vi "PathPlanner_Cmd_Follow_Internal_Replan_Sample.vi"(4 "PassthroughTime_SEC":dbl, 5 "Extra Time Sec":dbl, 6 "Reset In":bool, 7 "ReplanningConfig":T6={"enableInitialReplanning"=TRUE, "enableDynamicReplanning"=FALSE, "dynamicReplanningTotalErrorThreshold"=1.0, "dynamicReplanningErrorSpikeThreshold"=0.25}, 8 "Position Error M":dbl, 9 "Current Pose SI":T17 {"ROTATION"."SIN" format="%13.4f"; "ROTATION"."COS" format="%13.4f"; "ROTATION"."VALUE" format="%13.4f"; "TRANSLATION"."Y" format="%14.3f"; "TRANSLATION"."X" format="%14.3f"}, 10 "CurrentChassisSpeeds":T18 {"vOmega" format="%10.3f"; "vY" format="%10.3f"; "vX" format="%10.3f"}, 11 "RePlannedPath in":T11 {"AllPoints"."HolonomicRotation"."SIN" format="%13.4f"; "AllPoints"."HolonomicRotation"."COS" format="%13.4f"; "AllPoints"."HolonomicRotation"."VALUE" format="%13.4f"; "AllPoints"."Position"."Y" format="%14.3f"; "AllPoints"."Position"."X" format="%14.3f"; "GoalEndState"."Rotation"."SIN" format="%13.4f"; "GoalEndState"."Rotation"."COS" format="%13.4f"; "GoalEndState"."Rotation"."VALUE" format="%13.4f"; "RotationTargets"."target"."SIN" format="%13.4f"; "RotationTargets"."target"."COS" format="%13.4f"; "RotationTargets"."target"."VALUE" format="%13.4f"; "PreviewStartingRotation"."SIN" format="%13.4f"; "PreviewStartingRotation"."COS" format="%13.4f"; "PreviewStartingRotation"."VALUE" format="%13.4f"; "BezierPoints"."Y" format="%14.3f"; "BezierPoints"."X" format="%14.3f"}) -> (0 "Traj End Status":T5, 1 "Trajectory State":T7={"TimeSeconds"=0.0, "VelocityMPS"=0.0, "AccerationMpsSq"=0.0, "HeadingAngularVelRadPerSec"=0.0, "PositionMeters"={"X"=0.0, "Y"=0.0}, "Heading"={"VALUE"=0.0, "COS"=1.0, "SIN"=0.0}, "TargetHolonomicRotation"={"VALUE"=0.0, "COS"=1.0, "SIN"=0.0}, "CurvatureRadPerMeter"=0.0, "PathPlannerConstraints"={"MaxVelocityMps;"=0.0, "MaxAccelerationMpsSq;"=0.0, "MaxAngularVelRadPsEc;"=0.0, "MaxAngularAccRadPSecSq"=0.0, "Exists"=FALSE}, "DeltaPos"=0.0} {"TargetHolonomicRotation"."SIN" format="%13.4f"; "TargetHolonomicRotation"."COS" format="%13.4f"; "TargetHolonomicRotation"."VALUE" format="%13.4f"; "Heading"."SIN" format="%13.4f"; "Heading"."COS" format="%13.4f"; "Heading"."VALUE" format="%13.4f"; "PositionMeters"."Y" format="%14.3f"; "PositionMeters"."X" format="%14.3f"}, 2 "Reset Controller":bool, 3 "PathPlannerTrajectoryEvents":T1)   [LabVIEW 2019, in "PathPlanner24.lvlib"]
doc: "This is an internal function. It is not to be called by end users."
uses:
  PathPlanner24.lvlib
  <vilib>/Rock Robotics/WPI/ThirdParty/JAS_Junk/TrajLib/TypeDef/CHASSIS_SPEEDS.ctl
  TypeDef/PathPlannerPath.ctl
  <vilib>/Rock Robotics/WPI/ThirdParty/JAS_Junk/TrajLib/TypeDef/TRANSLATION2D.ctl
  <vilib>/Rock Robotics/WPI/ThirdParty/JAS_Junk/TrajLib/TypeDef/ROTATION2D.ctl
  TypeDef/PathPlannerRotationTarget.ctl
  TypeDef/PathPlannerConstraintsZone.ctl
  TypeDef/PathPlannerPathConstraints.ctl
  TypeDef/PathPlannerEventMarker.ctl
  TypeDef/PathPlannerCommandUtil.ctl
  ENum/PathPlanner_CommandUtilType_ENUM.ctl
  TypeDef/PathPlannerGoalEndState.ctl
  TypeDef/PathPlannerPathPoint.ctl
  <vilib>/Rock Robotics/WPI/ThirdParty/JAS_Junk/TrajLib/TypeDef/POSE2D.ctl
  TypeDef/PathPlannerTrajectoryState.ctl
  TypeDef/PathPlannerReplanningConfig.ctl
  <vilib>/Rock Robotics/WPI/ThirdParty/JAS_Junk/TrajLib/Rotation2d_GetDegrees.vi
  <vilib>/Rock Robotics/WPI/ThirdParty/JAS_Junk/TrajLib/MathUtil_InputModulus.vi
  <vilib>/Rock Robotics/WPI/ThirdParty/JAS_Junk/TrajLib/Rotation2d_CreateAngleDegrees.vi
  <vilib>/Rock Robotics/WPI/ThirdParty/JAS_Junk/TrajLib/Rotation2d_GetRadians.vi
  <vilib>/Rock Robotics/WPI/ThirdParty/JAS_Junk/TrajLib/Conv_Radians_Deg.vi
  <vilib>/Rock Robotics/WPI/ThirdParty/JAS_Junk/TrajLib/Conv_Deg_Radians.vi
  <vilib>/Rock Robotics/WPI/ThirdParty/JAS_Junk/TrajLib/Rotation2d_CreateAngle.vi
  <vilib>/Utility/semaphor.llb/Obtain Semaphore Reference.vi
  <vilib>/Rock Robotics/WPI/ThirdParty/JAS_Junk/TrajLib/Trajectory_Library.lvlib
  TypeDef/PathPlannerTrajectoryEvent.ctl
  TypeDef/PathPlannerTrajectoryEvents.ctl
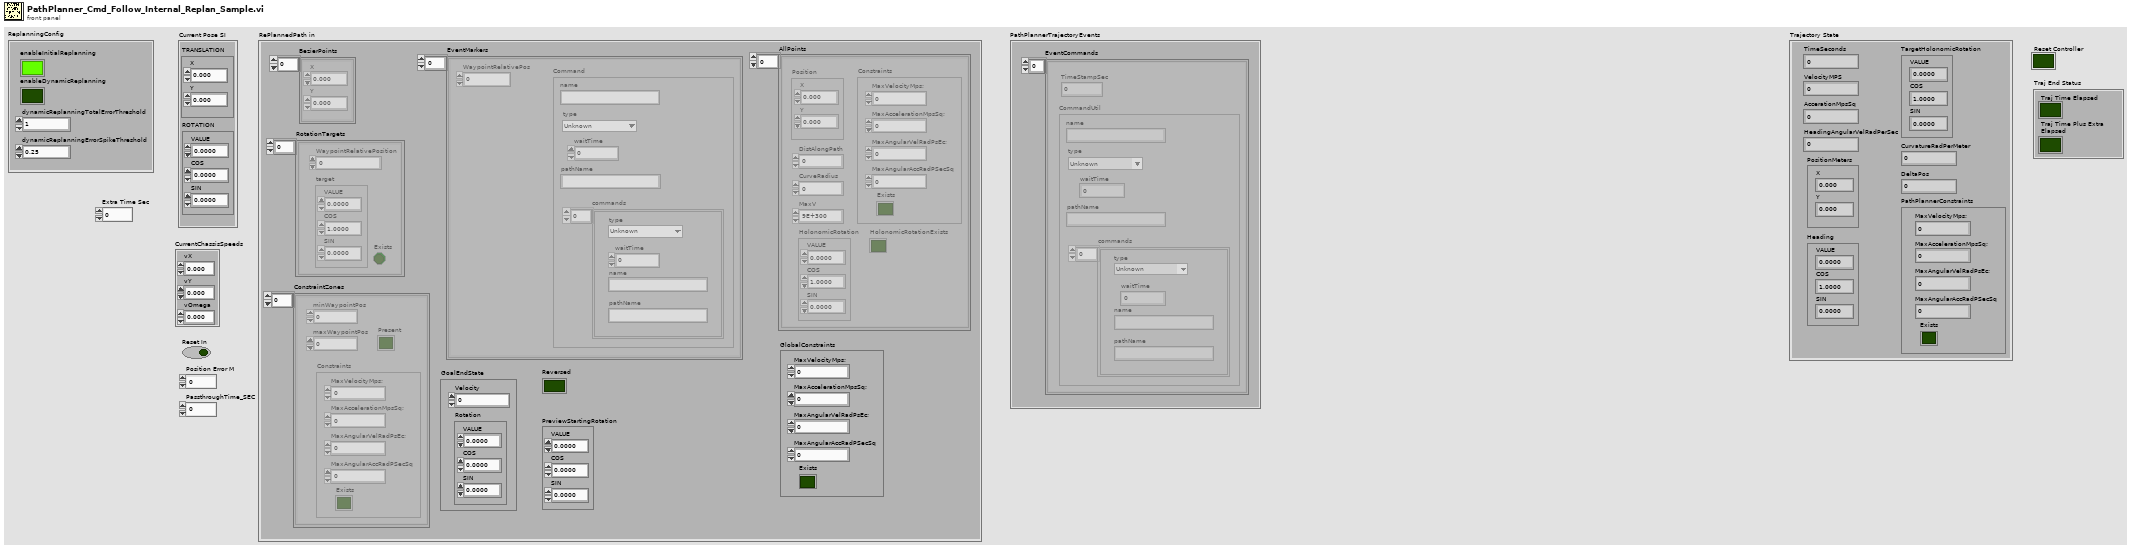
[diagram p1: front panel]
types:
  T1 = typedef "PathPlanner24.lvlib/PathPlannerTrajectoryEvents.ctl" = cluster{"EventCommands":T2[]}
  T2 = typedef "PathPlanner24.lvlib/PathPlannerTrajectoryEvent.ctl" = cluster{"TimeStampSec":dbl, "CommandUtil":T3}
  T3 = typedef "PathPlanner24.lvlib/PathPlannerCommandUtil.ctl" = cluster{"waitTime":dbl, "name":string, "pathName":string, "commands":cluster{"type":T4, "waitTime":dbl, "name":string, "pathName":string}[], "type":T4}
  T4 = typedef "PathPlanner24.lvlib/PathPlanner_CommandUtilType_ENUM.ctl" = enum16{"Unknown", "Wait", "Named", "Path", "Sequential", "Parallel", "Race", "Deadline"}
  T5 = cluster{"Traj Time Plus Extra\nElapsed":bool, "Traj Time Elapsed":bool}
  T6 = typedef "PathPlanner24.lvlib/PathPlannerReplanningConfig.ctl" = cluster{"enableInitialReplanning":bool, "enableDynamicReplanning":bool, "dynamicReplanningTotalErrorThreshold":dbl, "dynamicReplanningErrorSpikeThreshold":dbl}
  T7 = typedef "PathPlanner24.lvlib/PathPlannerTrajectoryState.ctl" = cluster{"TimeSeconds":dbl, "VelocityMPS":dbl, "AccerationMpsSq":dbl, "HeadingAngularVelRadPerSec":dbl, "PositionMeters":T8, "Heading":T9, "TargetHolonomicRotation":T9, "CurvatureRadPerMeter":dbl, "PathPlannerConstraints":T10, "DeltaPos":dbl}
  T8 = typedef "Trajectory_Library.lvlib/TRANSLATION2D.ctl" = cluster{"X":dbl, "Y":dbl}
  T9 = typedef "Trajectory_Library.lvlib/ROTATION2D.ctl" = cluster{"VALUE":dbl, "COS":dbl, "SIN":dbl}
  T10 = typedef "PathPlanner24.lvlib/PathPlannerPathConstraints.ctl" = cluster{"MaxVelocityMps;":dbl, "MaxAccelerationMpsSq;":dbl, "MaxAngularVelRadPsEc;":dbl, "MaxAngularAccRadPSecSq":dbl, "Exists":bool}
  T11 = typedef "PathPlanner24.lvlib/PathPlannerPath.ctl" = cluster{"BezierPoints":T8[], "PreviewStartingRotation":T9, "Reversed":bool, "RotationTargets":T12[], "ConstraintZones":T13[], "EventMarkers":T14[], "GlobalConstraints":T10, "GoalEndState":T15, "AllPoints":T16[]}
  T12 = typedef "PathPlanner24.lvlib/PathPlannerRotationTarget.ctl" = cluster{"target":T9, "WaypointRelativePosition":dbl, "Exists":bool}
  T13 = typedef "PathPlanner24.lvlib/PathPlannerConstraintsZone.ctl" = cluster{"minWaypointPos":dbl, "maxWaypointPos":dbl, "Constraints":T10, "Present":bool}
  T14 = typedef "PathPlanner24.lvlib/PathPlannerEventMarker.ctl" = cluster{"WaypointRelativePos":dbl, "Command":T3}
  T15 = typedef "PathPlanner24.lvlib/PathPlannerGoalEndState.ctl" = cluster{"Velocity":dbl, "Rotation":T9}
  T16 = typedef "PathPlanner24.lvlib/PathPlannerPathPoint.ctl" = cluster{"Position":T8, "HolonomicRotation":T9, "DistAlongPath":dbl, "CurveRadius":dbl, "MaxV":dbl, "Constraints":T10, "HolonomicRotationExists":bool}
  T17 = typedef "Trajectory_Library.lvlib/POSE2D.ctl" = cluster{"TRANSLATION":T8, "ROTATION":T9}
  T18 = typedef "Trajectory_Library.lvlib/CHASSIS_SPEEDS.ctl" = cluster{"vX":dbl, "vY":dbl, "vOmega":dbl}
  T19 = typedef "PathPlanner24.lvlib/PathPlannerTrajectory.ctl" = cluster{"States":T7[]}
  T20 = typedef "Trajectory_Library.lvlib/TIMER.ctl" = cluster{"StartTime":dbl, "Accumulated TIme":dbl, "Running":bool, "semaphore":T21}
  T21 = typedef "Semaphore RefNum" = refnum<k1>
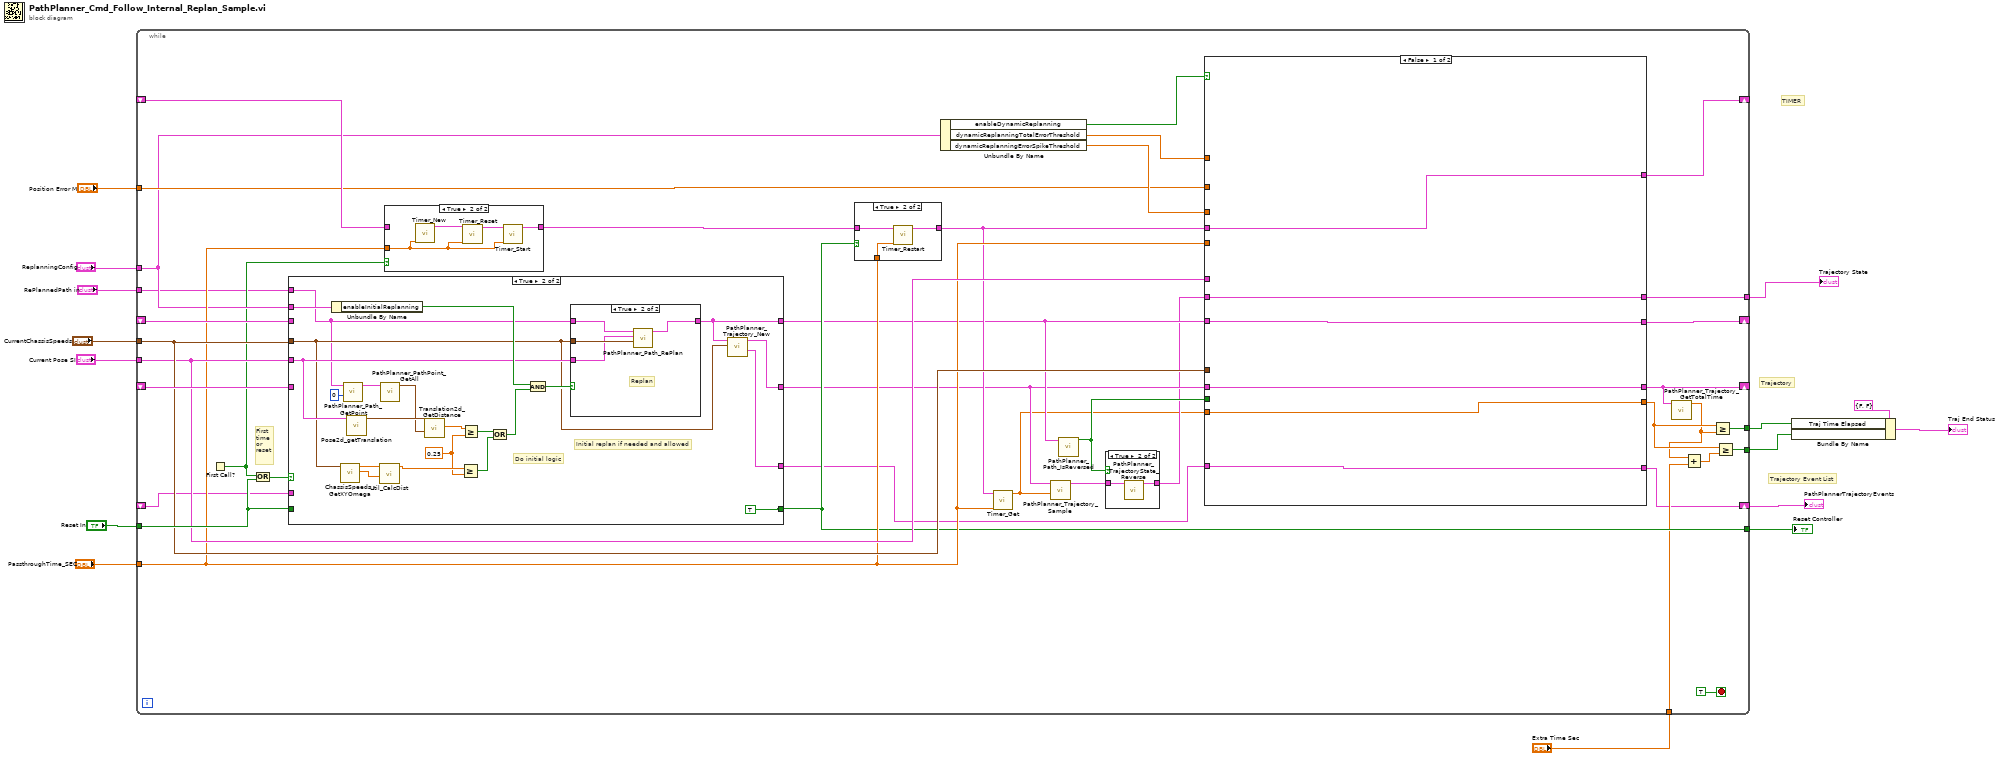
[diagram p0: block diagram]
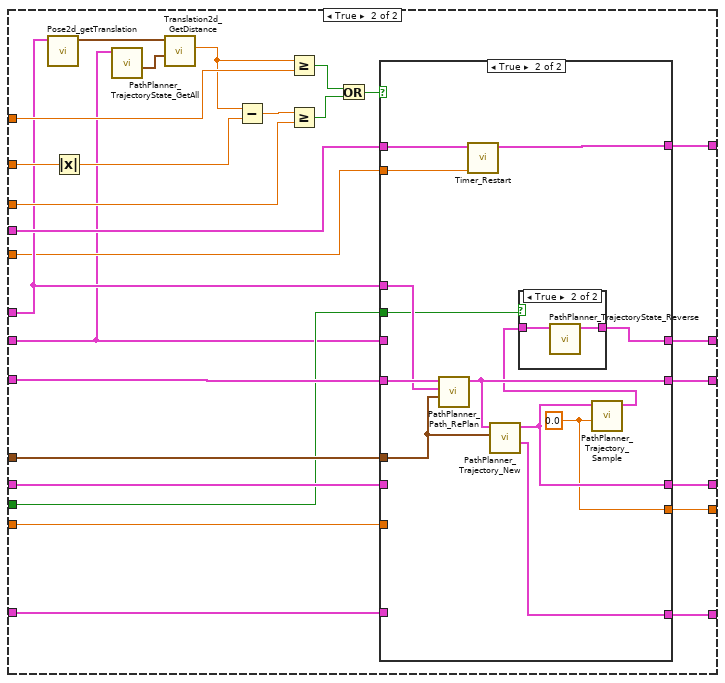
[diagram p2: hidden frame]
diagram:
  # "Trajectory Event List"
  # "TIMER"
  # "Trajectory"
  n1 = while {
    tunnel: "CurrentChassisSpeeds" -> [w48]
    tunnel: "Current Pose SI" -> [w47]
    shift-right: [w30] -> _
    shift-left: _ -> [w53]
    shift-right: [w37] -> _
    shift-left: _ -> [w52]
    tunnel: "Reset In" -> [w51]
    tunnel: [w36] -> w13
    tunnel: [w38] -> w11
    tunnel: "PassthroughTime_SEC" -> [w44]
    shift-right: [w32] -> _
    shift-left: _ -> [w45]
    tunnel: "Position Error M" -> [w35]
    tunnel: "ReplanningConfig" -> [w34]
    tunnel: [w29] -> w5
    tunnel: [w24] -> w4
    tunnel: "Extra Time Sec" -> [w23]
    shift-right: [w18] -> w1
    shift-left: _ -> [w17]
    tunnel: "RePlannedPath in" -> [w16]
    stop <- TRUE stop-if-true
    # "First\ntime\nor \nreset"
    n2 = First Call?() -> (First Call?: T/F=w31:bool)
    n3 = Or(x=w31, y=w51) -> (x .or. y?=w50:bool)
    n4 = case shown="True" w50 {
      tunnel: w52 -> [w123 _]
      tunnel: w48 -> [_ w130]
      tunnel: [w122 w129] -> w28
      tunnel: w34 -> [_ w145]
      tunnel: w47 -> [_ w131]
      tunnel: [w123 w128] -> w33
      tunnel: w53 -> [w122 _]
      tunnel: w51 -> [w124 _]
      tunnel: [w124 TRUE] -> w36
      tunnel: [w121 w126] -> w19
      tunnel: w17 -> [w121 _]
      tunnel: w16 -> [_ w125]
      frame False {
      }
      frame True {
        w133 = 0.25 ("y")
        # "Initial replan if needed and allowed"
        # "Do initial logic"
        n5 = Unbundle By Name(w145) -> ("enableInitialReplanning"=w138:bool)
        n6 = call <vilib>:"ChassisSpeeds_GetXYOmega.vi"("CHASSIS"=w130) -> ("vY"=w135:dbl, "vX"=w136:dbl)  [unwired: 8 in, 1 out]
        n7 = call "PathPlanner_Path_GetPoint.vi"("Index"=0, "PathPlannerPath"=w125) -> ("Point"=w143:T16)  [unwired: 9 in]
        n8 = call <vilib>:"Pose2d_getTranslation.vi"("in POSE"=w131) -> ("outTRANSLATION"=w144:T8)  [unwired: 10 in]
        n9 = call <vilib>:"Util_CalcDist.vi"("Y"=w135, "X"=w136) -> ("DIST"=w134:dbl)  [unwired: 9 in]
        n10 = call "PathPlanner_PathPoint_GetAll.vi"("PathPlannerPoint"=w143) -> ("Position"=w142:T8)  [unwired: 4 in, 6 out]
        n11 = call <vilib>:"Translation2d_GetDistance.vi"("other Translation"=w142, "In Translation"=w144) -> ("Distance"=w141:dbl)  [unwired: 9 in]
        n12 = Greater Or Equal?(x=w134, y=w133) -> (x >= y?=w132:bool)
        n13 = Greater Or Equal?(x=w141, y=w133) -> (x >= y?=w140:bool)
        n14 = Or(x=w140, y=w132) -> (x .or. y?=w139:bool)
        n15 = And(x=w138, y=w139) -> (x .and. y?=w137:bool)
        n16 = case shown="True" w137 {
          tunnel: w125 -> [w147 w151]
          tunnel: w130 -> [_ w150]
          tunnel: w131 -> [_ w149]
          tunnel: [w147 w148] -> w128
          frame False {
          }
          frame True {
            # "Replan"
            n17 = call "PathPlanner_Path_RePlan.vi"("CurrentSpeeds"=w150, "StartingPose"=w149, "in PathPlannerPath"=w151) -> ("RePlannedPath"=w148:T11)  [unwired: 7 in, 1 out]
          }
        }
        n18 = call "PathPlanner_Trajectory_New.vi"("StartingSpeeds"=w130, "Path"=w128) -> ("PathPlannerTrajectoryEvents"=w126:T1, "PathPlannerTrajectory"=w129:T19)  [unwired: 8 in]
      }
    }
    n19 = case shown="True" w31 {
      tunnel: w44 -> [_ w118]
      tunnel: [w116 w117] -> w46
      tunnel: w45 -> [w116 _]
      frame False {
      }
      frame True {
        n20 = call <vilib>:"Timer_New.vi"("Pass_Through_Time"=w118) -> ("TIMER"=w120:T20)  [unwired: 10 in]
        n21 = call <vilib>:"Timer_Reset.vi"("Pass_Through_Time"=w118, "in TIMER"=w120) -> ("out TIMER"=w119:T20)  [unwired: 9 in]
        n22 = call <vilib>:"Timer_Start.vi"("Pass_Through_Time"=w118, "in Timer"=w119) -> ("out Timer"=w117:T20)  [unwired: 9 in]
      }
    }
    n23 = case shown="True" w36 {
      tunnel: w46 -> [w109 w112]
      tunnel: [w109 w111] -> w41
      tunnel: w44 -> [_ w110]
      frame False {
      }
      frame True {
        n24 = call <vilib>:"Timer_Restart.vi"("Pass_Through_Time"=w110, "in Timer"=w112) -> ("out Timer"=w111:T20)  [unwired: 9 in]
      }
    }
    n25 = Unbundle By Name(w34) -> ("enableDynamicReplanning"=w40:bool, "dynamicReplanningTotalErrorThreshold"=w42:dbl, "dynamicReplanningErrorSpikeThreshold"=w43:dbl)
    n26 = call <vilib>:"Timer_Get.vi"("Pass_Through_Time"=w44, "TIMER"=w41) -> ("CurrentTImer"=w20:dbl)  [unwired: 9 in]
    n27 = call "PathPlanner_Trajectory_Sample.vi"("Time"=w20, "PathPlannerTrajectory"=w28) -> ("PathPlannerState"=w39:T7)  [unwired: 9 in]
    n28 = call "PathPlanner_Path_IsReversed.vi"("PathPlannerPath"=w33) -> ("Reversed"=w22:bool)  [unwired: 10 in]
    n29 = case shown="True" w22 {
      tunnel: w39 -> [w113 w115]
      tunnel: [w113 w114] -> w21
      frame False {
      }
      frame True {
        n30 = call "PathPlanner_TrajectoryState_Reverse.vi"("PathPlannerState"=w115) -> ("Reversed State"=w114:T7)  [unwired: 10 in]
      }
    }
    n31 = case shown="False" w40 {
      tunnel: w35 -> [_ w86]
      tunnel: w41 -> [w59 w77]
      tunnel: [w59 w76] -> w32
      tunnel: w47 -> [_ w73]
      tunnel: w42 -> [_ w83]
      tunnel: w43 -> [_ w79]
      tunnel: [w57 w75] -> w37
      tunnel: [w56 w74] -> w38
      tunnel: w48 -> [_ w72]
      tunnel: w28 -> [w58 w71]
      tunnel: [w58 w70] -> w30
      tunnel: w44 -> [_ w67]
      tunnel: w33 -> [w57 w66]
      tunnel: [w55 w65] -> w27
      tunnel: w22 -> [_ w64]
      tunnel: w21 -> [w56 w63]
      tunnel: w20 -> [w55 w62]
      tunnel: w19 -> [w54 w61]
      tunnel: [w54 w60] -> w18
      frame False {
      }
      frame True {
        n32 = call <vilib>:"Pose2d_getTranslation.vi"("in POSE"=w73) -> ("outTRANSLATION"=w84:T8)  [unwired: 10 in]
        n33 = Absolute Value(x=w86) -> (abs(x)=w82:dbl)
        n34 = call "PathPlanner_TrajectoryState_GetAll.vi"("PathPlannerState"=w63) -> ("PositionMeters"=w85:T8)  [unwired: 1 in, 9 out]
        n35 = call <vilib>:"Translation2d_GetDistance.vi"("other Translation"=w85, "In Translation"=w84) -> ("Distance"=w81:dbl)  [unwired: 9 in]
        n36 = Subtract(x=w81, y=w82) -> (x-y=w80:dbl)
        n37 = Greater Or Equal?(x=w81, y=w83) -> (x >= y?=w68:bool)
        n38 = Greater Or Equal?(x=w80, y=w79) -> (x >= y?=w69:bool)
        n39 = Or(x=w68, y=w69) -> (x .or. y?=w78:bool)
        n40 = case shown="True" w78 {
          tunnel: w77 -> [w92 w105]
          tunnel: [w92 w104] -> w76
          tunnel: w66 -> [w91 w103]
          tunnel: [w91 w101] -> w75
          tunnel: w63 -> [w90 _]
          tunnel: [w90 w97] -> w74
          tunnel: w73 -> [_ w102]
          tunnel: w72 -> [_ w100]
          tunnel: w71 -> [w89 _]
          tunnel: [w89 w99] -> w70
          tunnel: w64 -> [_ w96]
          tunnel: w67 -> [_ w95]
          tunnel: [w88 w94] -> w65
          tunnel: w62 -> [w88 _]
          tunnel: w61 -> [w87 _]
          tunnel: [w87 w93] -> w60
          frame False {
          }
          frame True {
            w94 = 0.0 ("Time")
            n41 = call "PathPlanner_Path_RePlan.vi"("CurrentSpeeds"=w100, "StartingPose"=w102, "in PathPlannerPath"=w103) -> ("RePlannedPath"=w101:T11)  [unwired: 7 in, 1 out]
            n42 = call <vilib>:"Timer_Restart.vi"("Pass_Through_Time"=w95, "in Timer"=w105) -> ("out Timer"=w104:T20)  [unwired: 9 in]
            n43 = call "PathPlanner_Trajectory_New.vi"("StartingSpeeds"=w100, "Path"=w101) -> ("PathPlannerTrajectoryEvents"=w93:T1, "PathPlannerTrajectory"=w99:T19)  [unwired: 8 in]
            n44 = call "PathPlanner_Trajectory_Sample.vi"("Time"=w94, "PathPlannerTrajectory"=w99) -> ("PathPlannerState"=w98:T7)  [unwired: 9 in]
            n45 = case shown="True" w96 {
              tunnel: w98 -> [w106 w108]
              tunnel: [w106 w107] -> w97
              frame False {
              }
              frame True {
                n46 = call "PathPlanner_TrajectoryState_Reverse.vi"("PathPlannerState"=w108) -> ("Reversed State"=w107:T7)  [unwired: 10 in]
              }
            }
          }
        }
      }
    }
    n47 = call "PathPlanner_Trajectory_GetTotalTime.vi"("PathPlannerTrajectory"=w30) -> ("TotalTimeSeconds"=w25:dbl)  [unwired: 10 in]
    n48 = Add(x=w25, y=w23) -> (x+y=w26:dbl)
    n49 = Greater Or Equal?(x=w27, y=w25) -> (x >= y?=w29:bool)
    n50 = Greater Or Equal?(x=w27, y=w26) -> (x >= y?=w24:bool)
  }
  "Reset Controller" <- w13
  "Trajectory State" <- w11
  "PathPlannerTrajectoryEvents" <- w1
  n51 = Bundle By Name(cluster=T5 {"Traj Time Plus Extra\nElapsed"=FALSE, "Traj Time Elapsed"=FALSE} ("Traj End Status"), "Traj Time Elapsed"=w5, "Traj Time Plus Extra\nElapsed"=w4) -> (→"Traj End Status":T5)
